vi "Launch PID.vi"(8 "error in (no error)":errorcluster, 11 "Baratron in":refnum<class "Baratron.lvclass">) -> (0 "error out":errorcluster, 3 "Baratron out":refnum<class "Baratron.lvclass">)   [LabVIEW 2021]
uses:
  <vilib>/MGI/Panel Manager/Panel Actor/Panel Actor/Panel Actor.lvclass
  <vilib>/MGI/Panel Manager/Panel/Panel.lvlib
  <vilib>/MGI/Panel Manager/Panel/Panel/Subpanel/Subpanel.vi
  <vilib>/MGI/Panel Manager/Panel/Panel/Subpanel/Subpanel.lvclass
  PID-Ctl/PID Ctl/PID Ctl.lvclass
  PID-Ctl/PID Ctl/Config Data.ctl
  Baratron.lvclass
  C:/Program Files/National Instruments/LabVIEW 2021/vi.lib/MGI/Panel Manager/Panel Actor/Panel Actor/Panel Actor.lvclass
  C:/Program Files/National Instruments/LabVIEW 2021/vi.lib/ActorFramework/Actor/Actor.lvclass
  C:/PPLs/Baratron/Baratron/Baratron.lvclass
  C:/PPLs/DAQ-arch/DAQ/AI Interface/AI Interface/AI Interface.lvclass
  C:/Program Files/National Instruments/LabVIEW 2021/vi.lib/MGI/Panel Manager/Panel/Panel/Panel.lvclass
  C:/Program Files/National Instruments/LabVIEW 2021/vi.lib/MGI/Panel Manager/Panel/Panel/Subpanel/Subpanel.lvclass
  C:/PPLs/PID-Ctl/PID Ctl/PID Ctl.lvclass
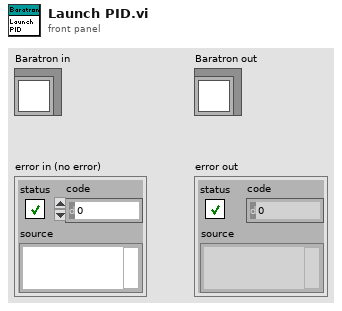
[diagram p1: front panel]
types:
  T1 = typedef "PID Ctl.lvlib/PID Ctl.lvclass/Config Data.ctl" = cluster{"Loop Timing (ms)":u32}
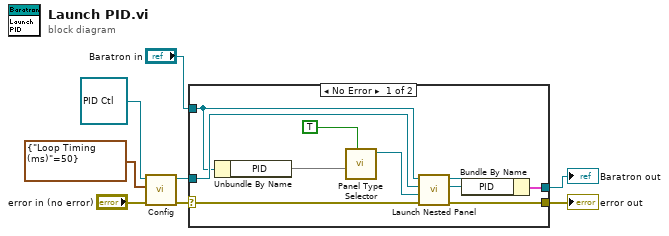
[diagram p0: block diagram]
diagram:
  n1 = call "Config.vi"("error in (no error)"="error in (no error)", "Config Data"=T1 {"Loop Timing (ms)"=50}, "PID Ctl in"=refnum<class "PID Ctl.lvclass"> refnum ("PID Ctl.lvlib:PID Ctl.lvclass")) -> ("error out"=w8:errorcluster, "PID Ctl out"=w6:refnum<class "PID Ctl.lvclass">)  [unwired: 7 in]
  n2 = case shown="No Error" w8 {
    selector: w8 -> [w11 w19]
    tunnel: "Baratron in" -> [w10 w20]
    tunnel: [w16 w20] -> w3
    tunnel: [w14 w19] -> w1
    tunnel: w6 -> [w12 _]
    frame No Error {
      n3 = Unbundle By Name(w10) -> ("PID"=w9)
      n4 = call-poly <vilib>:"Panel Type Selector.vi"("Autoshow? (T)"=TRUE, "Sub Panel"=w9) -> ("Subpanel Out"=w17:refnum<class "Subpanel.lvclass">)  [unwired: 8 in, 1 out]
      n5 = call <vilib>:"Launch Nested Panel.vi"("error in (no error)"=w11, "Panel"=w17, "Nested Panel Actor"=w12, "Panel Actor in"=w10) -> ("error out"=w14:errorcluster, "Nested Actor's Enqueuer"=w15:refnum<class "Message Enqueuer.lvclass">, "Panel Actor out"=w18:refnum<class "Baratron.lvclass">)  [unwired: 4 in, 1 out]
      n6 = Bundle By Name(cluster=w18, "PID"=w15) -> (w16:cluster{})
    }
    frame Error {
    }
  }
  "error out" <- w1
  "Baratron out" <- w3
